vi "CALC_TRAN_TIME_LPFREQ.vi"(0 "VISA IN":refnum<visa-resource-name>, 5 "error in":errorcluster, 7 "Channel":i32) -> (14 "VISA Out":refnum<visa-resource-name>, 19 "error out":errorcluster)   [LabVIEW 2018, in "PNA-X.lvlib"]
doc: "CALCulate<cnum>:TRANsform:TIME:LPFREQuency \n1568\n\n(Write-only) Sets the start frequencies in LowPass Mode. \nSee Critical Note \nParameters \n<cnum> Channel number of the measurement. There must be a selected measurement \non that channel. If unspecified, <cnum> is set to 1. \nExamples CALC:TRAN:TIME:LPFR \ncalculate2:transform:time:lpfrequency \nQuery Syntax Not applicable \nDefault Not applicable"
uses:
  PNA-X.lvlib
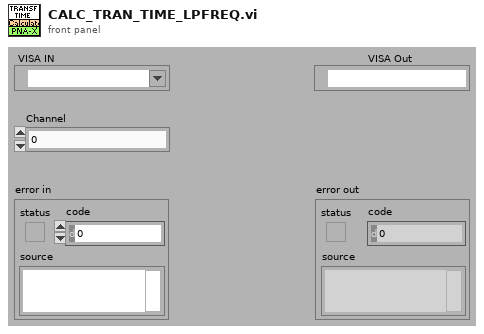
[diagram p1: front panel]
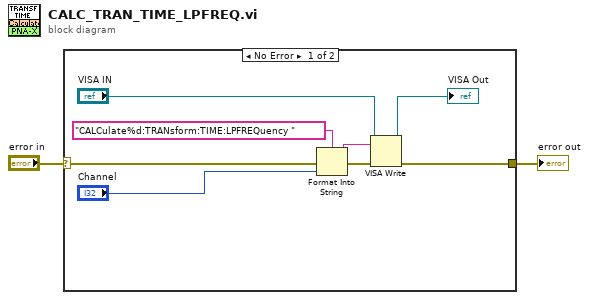
[diagram p0: block diagram]
diagram:
  n1 = case shown="No Error" "error in" {
    selector: "error in" -> [w10 w11]
    tunnel: [w5 w11] -> w1
    frame No Error {
      n2 = Format Into String(format string="CALCulate%d:TRANsform:TIME:LPFREQuency " ("Cmdline"), error in=w10, "Channel") -> (resulting string=w8:string, error out=w9:errorcluster)  [unwired: 1 in]
      n3 = VISA Write(VISA resource name="VISA IN", write buffer=w8, error in (no error)=w9) -> (VISA resource name out=→"VISA Out":refnum<visa-resource-name>, error out=w5:errorcluster)  [unwired: 1 out]
    }
    frame Error {
    }
  }
  "error out" <- w1
